vi "Create.vi"(7 "user interface type":T3, 8 "error in (no error)":errorcluster, 9 "component settings":T1[](array[typedef]), 10 "Components":refnum<class "Component.lvclass">[](array[class]), 11 "Component Settings Editor in":refnum<class "Component Settings Editor.lvclass">) -> (0 "error out":errorcluster, 3 "Component Settings Editor out":refnum<class "Component Settings Editor.lvclass">)   [LabVIEW 2017, in "DSF Core.lvlib" / "Component Settings Editor.lvclass"]
uses:
  Component Settings Editor.lvclass
  Component/Component.lvclass
  Component User Interface/UI Type.ctl
  Typedefs/DSF Settings Info.ctl
  Typedefs/DSF Version Info.ctl
  Component Settings Editor.lvclass/Component Settings Editor.ctl
  Component User Interface/Component User Interfaces.lvclass
  User Interface.lvclass
  DSF Core.lvlib
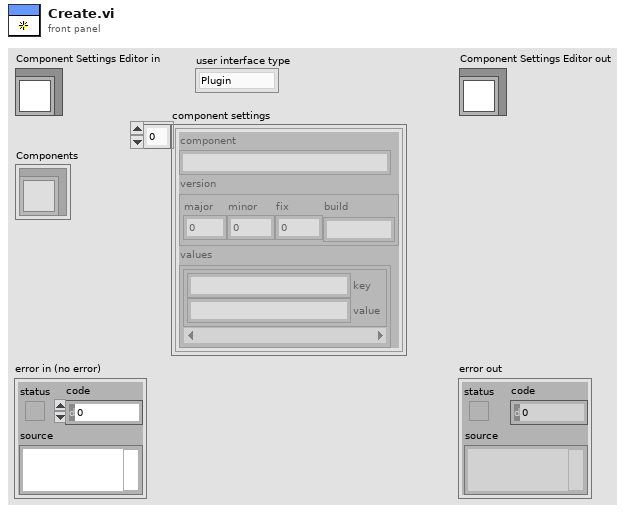
[diagram p1: front panel]
types:
  T1 = typedef "DSF Core.lvlib/DSF Settings Info.ctl" = cluster{"component":string, "version":T2, "values":cluster{"key":string, "value":string}[]}
  T2 = typedef "DSF Core.lvlib/DSF Version Info.ctl" = cluster{"major":u32, "minor":u32, "fix":u32, "build":string}
  T3 = typedef "DSF Core.lvlib/Component User Interfaces.lvclass/UI Type.ctl" = enum16{"Plugin", "Thread", "Rx Group", "Tx Group", "Rx Transfer", "Tx Transfer", "Rx Channel", "Tx Channel"}
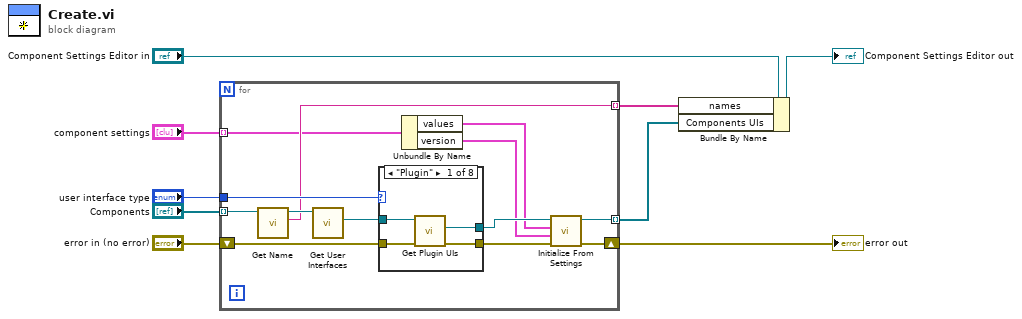
[diagram p0: block diagram]
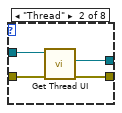
[diagram p2: hidden frame]
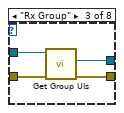
[diagram p3: hidden frame]
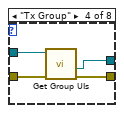
[diagram p4: hidden frame]
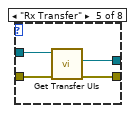
[diagram p5: hidden frame]
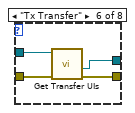
[diagram p6: hidden frame]
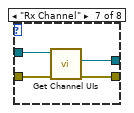
[diagram p7: hidden frame]
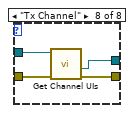
[diagram p8: hidden frame]
diagram:
  n1 = for {
    tunnel: "Components" -> [w22] mode=indexing
    tunnel: [w17] -> w6 mode=indexing
    tunnel: [w11] -> w2 mode=indexing
    tunnel: "user interface type" -> [w19]
    shift-right: [w10] -> w3
    shift-left: "error in (no error)" -> [w18]
    tunnel: "component settings" -> [w12] mode=indexing
    n2 = call "Get Name.vi"("Component in"=w22) -> ("name"=w17:string, "Component out"=w21:refnum<class "Component.lvclass">)  [unwired: 9 in]
    n3 = call "Get User Interfaces.vi"("Component in"=w21) -> ("User Interfaces"=w20:refnum<class "Component User Interfaces.lvclass">)  [unwired: 9 in, 1 out]
    n4 = case shown="\"Plugin\"" w19 {
      tunnel: [w26 w30 w34 w37 w42 w45 w47 w51] -> w15
      tunnel: w20 -> [w25 w29 w33 w38 w41 w46 w50 w54]
      tunnel: [w24 w27 w31 w35 w39 w43 w48 w52] -> w16
      tunnel: w18 -> [w23 w28 w32 w36 w40 w44 w49 w53]
      frame "Plugin" {
        n5 = call "Get Plugin UIs.vi"("error in (no error)"=w23, "Component UI in"=w25) -> ("error out"=w24:errorcluster, "Plugin Settings UI"=w26:refnum<class "User Interface.lvclass">)  [unwired: 7 in, 1 out]
      }
      frame "Thread" {
        n6 = call "Get Thread UI.vi"("error in (no error)"=w28, "Component UI in"=w29) -> ("error out"=w27:errorcluster, "Thread Settings UI"=w30:refnum<class "User Interface.lvclass">)  [unwired: 7 in, 1 out]
      }
      frame "Rx Group" {
        n7 = call "Get Group UIs.vi"("error in (no error)"=w32, "Component UI in"=w33) -> ("error out"=w31:errorcluster, "Rx Group UI"=w34:refnum<class "User Interface.lvclass">)  [unwired: 6 in, 2 out]
      }
      frame "Tx Group" {
        n8 = call "Get Group UIs.vi"("error in (no error)"=w36, "Component UI in"=w38) -> ("error out"=w35:errorcluster, "Tx Group UI"=w37:refnum<class "User Interface.lvclass">)  [unwired: 6 in, 2 out]
      }
      frame "Rx Transfer" {
        n9 = call "Get Transfer UIs.vi"("error in (no error)"=w40, "Component UI in"=w41) -> ("error out"=w39:errorcluster, "Rx Transfer UI"=w42:refnum<class "User Interface.lvclass">)  [unwired: 6 in, 2 out]
      }
      frame "Tx Transfer" {
        n10 = call "Get Transfer UIs.vi"("error in (no error)"=w44, "Component UI in"=w46) -> ("error out"=w43:errorcluster, "Tx Transfer UI"=w45:refnum<class "User Interface.lvclass">)  [unwired: 6 in, 2 out]
      }
      frame "Rx Channel" {
        n11 = call "Get Channel UIs.vi"("error in (no error)"=w49, "Component UI in"=w50) -> ("error out"=w48:errorcluster, "Rx Channel UI"=w47:refnum<class "User Interface.lvclass">)  [unwired: 6 in, 2 out]
      }
      frame "Tx Channel" {
        n12 = call "Get Channel UIs.vi"("error in (no error)"=w53, "Component UI in"=w54) -> ("error out"=w52:errorcluster, "Tx Channel UI"=w51:refnum<class "User Interface.lvclass">)  [unwired: 6 in, 2 out]
      }
    }
    n13 = Unbundle By Name(w12) -> ("values"=w13:cluster{"key":string, "value":string}[], "version"=w14:T2)
    n14 = call "Initialize From Settings.vi"("error in (no error)"=w16, "settings version"=w14, "settings"=w13, "User Interface in"=w15) -> ("error out"=w10:errorcluster, "User Interface out"=w11:refnum<class "User Interface.lvclass">)  [unwired: 6 in]
  }
  "error out" <- w3
  n15 = Bundle By Name(cluster="Component Settings Editor in", "names"=w6, "Components UIs"=w2) -> (→"Component Settings Editor out":refnum<class "Component Settings Editor.lvclass">)
